vi "Clear.vi"(8 "error in (no error)":errorcluster, 11 "Mock Process In":refnum<class "Mock Process.lvclass">) -> (0 "error out":errorcluster)   [LabVIEW 2020, in "Mock Process.lvclass"]
doc: "Clears any resorces allocated during initialization."
uses:
  Mock Process.lvclass
  Mock Process.lvclass/Mock Process.ctl
  Framework/Process/Process.lvclass
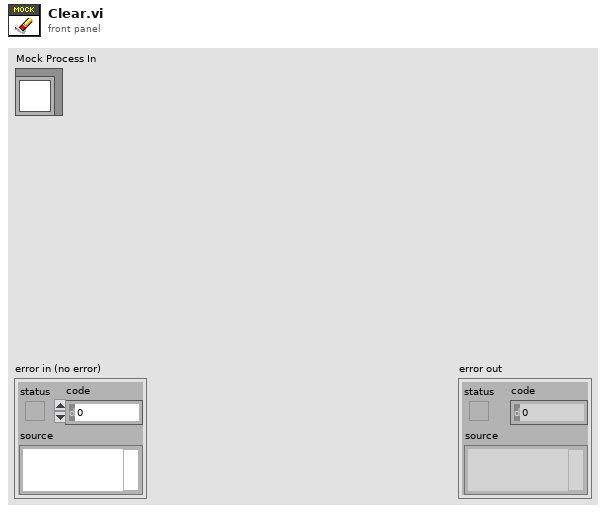
[diagram p1: front panel]
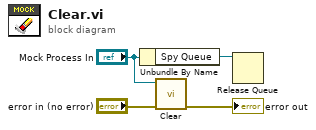
[diagram p0: block diagram]
diagram:
  n1 = Unbundle By Name("Mock Process In") -> ("Spy Queue"=w3:refnum<queue>)
  n2 = call-parent "Clear.vi"("error in (no error)"="error in (no error)", "Process In"="Mock Process In") -> ("error out"=→"error out":errorcluster)  [unwired: 9 in]
  n3 = Release Queue(queue=w3) -> ()  [unwired: 2 in, 3 out]
